vi "Button and Switch CCS.vi"() -> ()   [LabVIEW 2020]
uses:
  <vilib>/addons/control/pid/autopid.llb/PID autotuning parameters (adv).ctl
  <vilib>/addons/control/pid/pid.llb/PID Time Unit.ctl
  <vilib>/addons/control/pid/pid.llb/PID Structure.ctl
  <vilib>/addons/control/pid/pid.llb/PID Gain Unit.ctl
  <vilib>/Instr/_visa.llb/VISA Configure Serial Port (Instr).vi
  <vilib>/addons/control/pid/pid.llb/PID Structure Conversion (DBL).vi
  <vilib>/addons/control/pid/pid.llb/PID Advanced (DBL).vi
  <vilib>/addons/control/pid/NI_PID_autopid.lvlib
  <vilib>/ptbypt/NI_PtbyPt.lvlib
  <vilib>/addons/control/pid/NI_PID_pid.lvlib
panel:
  out "PWM Previous":dbl
  in  "auto? ACC":bool=TRUE
  out "Limit Setpoint":u64
  out "Limit Active":bool
  in  "Limit -":bool
  in  "Limit +":bool
  in  "Limit Speed":bool
  in  "gamma":dbl format="%.2f"
  in  "alpha":dbl=0.2 format="%.2f"
  in  "proportional unit":T1 items=["Gain (K)", "Band (PB)"]
  in  "PID structure":T2 items=["Academic (Standard)", "Parallel", "Series"]
  in  "derivative unit":T3=1 items=["min", "s"]
  in  "integral unit":T3=1 items=["min", "s"]
  in  "derivative":dbl
  in  "integral":dbl
  in  "proportional":dbl=10.0
  in  "linearity":dbl=0.9 format="%.2f"
  in  "beta":dbl=0.7 format="%.2f"
  in  "reinitialize? (F) 2":bool
  out "Speed Setpoint (km/h)":dbl
  out "Target Distance (m)":dbl
  out "Time Level":dbl=1.0
  out "Distance (m)":i8=73
  out "Brake Light":bool
  in  "VISA resource name":refnum<visa-resource-name>="COM15"
  in  "baud rate":u32=115200
  out "RPM":i64(knob) scale=0.0..650.0
  out "VELOCITY":u64(knob) scale=0.0..200.0
  out "GAS PEDAL":u8(slide)=1 scale=0.0..255.0
  out "BRAKE PEDAL":u8(slide)=1 scale=0.0..255.0
  out "VELOCITY":cluster{"VELOCITY":u64, "Cruise Setpoint":u64}(graph)
  in  "autotune? (F)":bool
  in  "PID gains":T4={"proportional gain (Kc)"=0.261831, "integral time (Ti, min)"=0.013639, "derivative time (Td, min)"=0.0} {"derivative time (Td, min)" format="%#.6g"; "integral time (Ti, min)" format="%#.6g"; "proportional gain (Kc)" format="%#.6g"}
  in  "dt (s)":dbl=0.02
  in  "reinitialize? (F)":bool
  in  "autotuning parameters":T5={"technique"=0, "type of controller"=1, "control specification"=0, "amplitude"=30.0} {"amplitude" format="%.2f"; "control specification" items=["normal", "fast", "slow"]; "type of controller" items=["P", "PI", "PID"]; "technique" items=["Step Open Loop", "Step Closed Loop", "Relay", "PID Relay"]}
  out "completed?":bool
  out "tuned PID gains":T4={"proportional gain (Kc)"=0.664899, "integral time (Ti, min)"=0.008397, "derivative time (Td, min)"=0.0} {"derivative time (Td, min)" format="%#.6g"; "integral time (Ti, min)" format="%#.6g"; "proportional gain (Kc)" format="%#.6g"}
  in  "auto? Speed Control":bool
  in  "ACCEPT SPEED PID":bool
  out "MOTOR CONTROL":dbl(graph)=1.0
  in  "stop":bool
  in  "PID Mode":i64(knob)=1 scale=1.0..3.0
  in  "Cruise Enable":bool
  in  "Distance":bool
  out "Distance Level":i8=1
  out "Cruise Active":bool
  out "Cruise Setpoint":u64
  in  "Speed +":bool
  in  "Speed -":bool
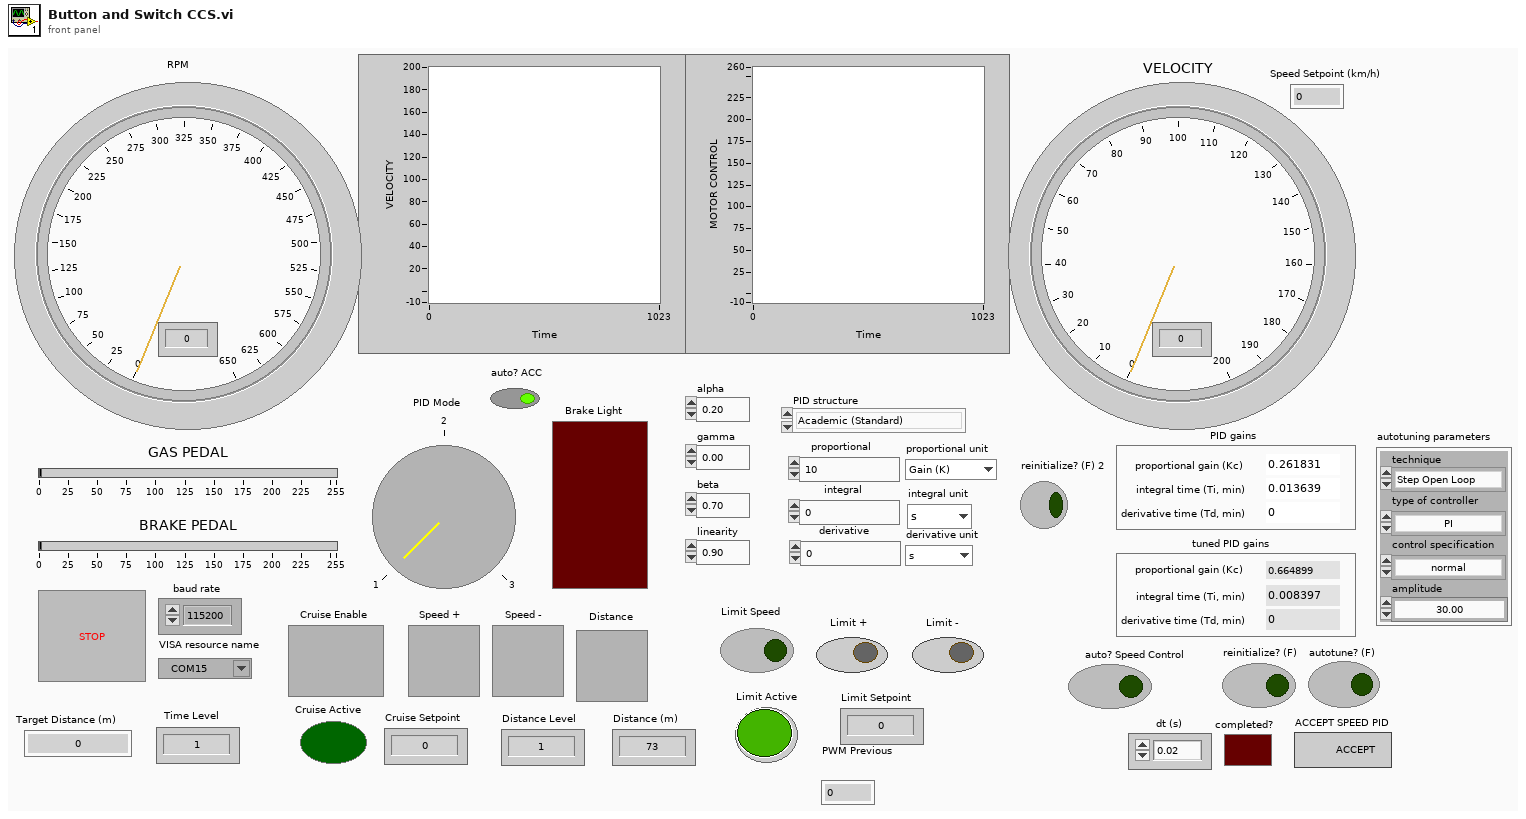
[diagram p1: front panel]
types:
  T1 = typedef "NI_PID_pid.lvlib/PID Gain Unit.ctl" = u16
  T2 = typedef "NI_PID_pid.lvlib/PID Structure.ctl" = u16
  T3 = typedef "NI_PID_pid.lvlib/PID Time Unit.ctl" = u16
  T4 = cluster{"proportional gain (Kc)":dbl, "integral time (Ti, min)":dbl, "derivative time (Td, min)":dbl}
  T5 = typedef "NI_PID_autopid.lvlib/PID autotuning parameters (adv).ctl" = cluster{"technique":u16, "type of controller":u16, "control specification":u16, "amplitude":dbl}
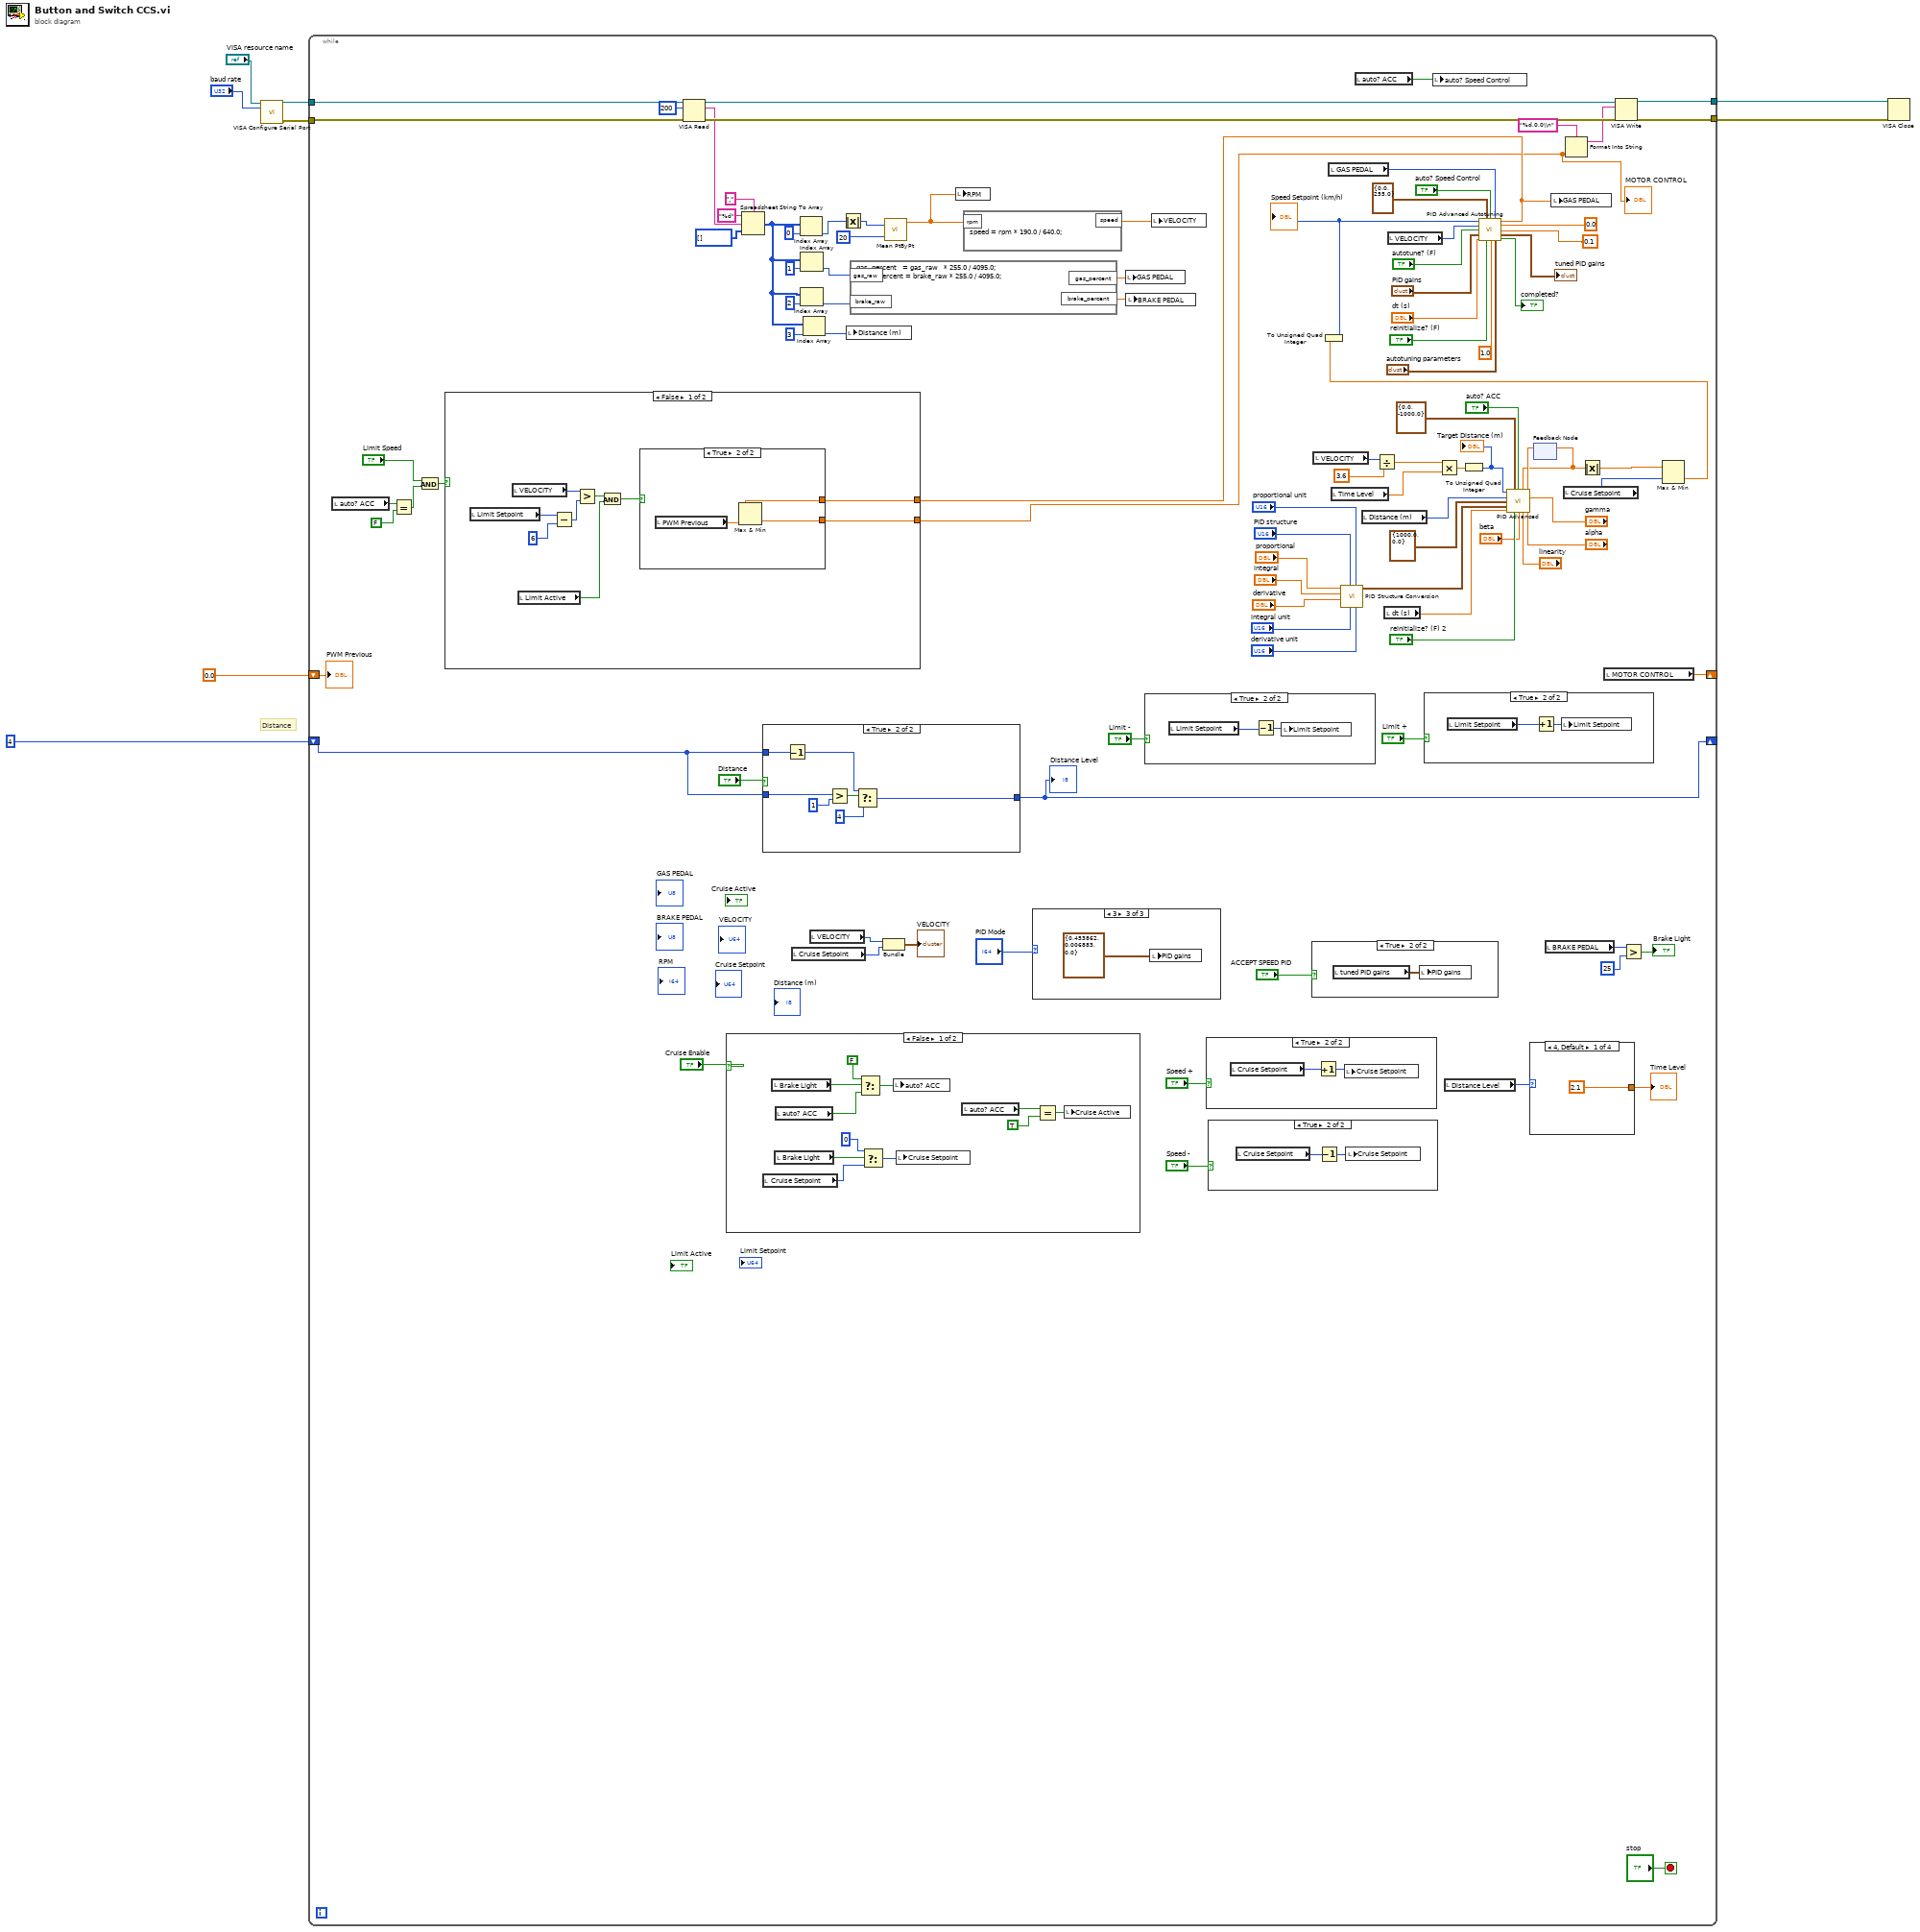
[diagram p0: block diagram]
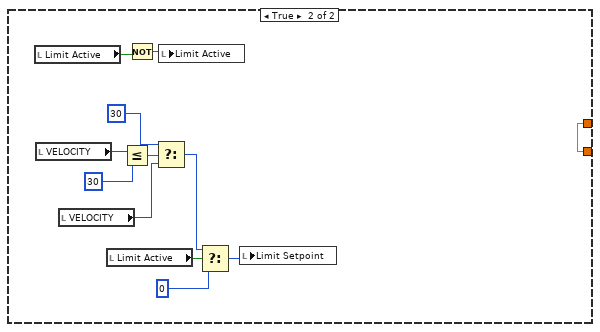
[diagram p5: hidden frame]
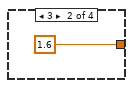
[diagram p6: hidden frame]
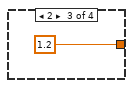
[diagram p7: hidden frame]
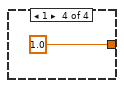
[diagram p8: hidden frame]
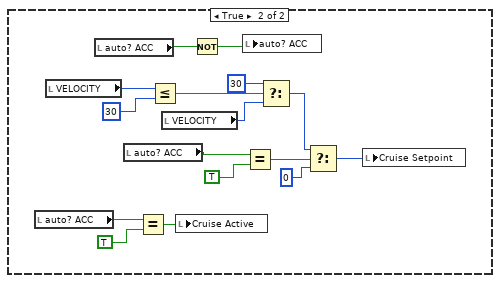
[diagram p12: hidden frame]
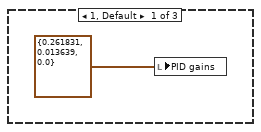
[diagram p13: hidden frame]
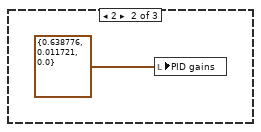
[diagram p14: hidden frame]
diagram:
  # "Distance"
  n1 = call-poly "VISA Configure Serial Port"("VISA resource name"="VISA resource name", "baud rate (9600)"="baud rate") -> ("VISA resource name out"=w7:refnum<visa-resource-name>, "error out"=w6:errorcluster)  [unwired: 12 in]
  n2 = while {
    tunnel: w7 -> [w109]
    tunnel: w6 -> [w108]
    tunnel: [w83] -> w5
    tunnel: [w84] -> w4
    shift-right: [w60] -> _
    shift-left: i64 4 ("f") -> [w61]
    shift-right: [w15] -> _
    shift-left: 0.0 ("MOTOR CONTROL") -> [w13]
    stop <- "stop" stop-if-true
    n3 = local read "auto? ACC"() -> (w20:bool)
    n4 = Equal?(x=w20, y=FALSE) -> (x = y?=w19:bool)
    n5 = And(x="Limit Speed", y=w19) -> (x .and. y?=w12:bool)
    n6 = VISA Read(VISA resource name=w109, byte count=u32 200, error in (no error)=w108) -> (VISA resource name out=w106:refnum<visa-resource-name>, read buffer=w104:string, error out=w107:errorcluster)  [unwired: 1 out]
    n7 = case shown="False" "Cruise Enable" {
      frame False {
        n8 = local read "Cruise Setpoint"() -> (w157:u64)
        n9 = local read "Brake Light"() -> (w165:bool)
        n10 = local read "Brake Light"() -> (w158:bool)
        n11 = local read "auto? ACC"() -> (w162:bool)
        n12 = Select(t=FALSE, s=w165, f=w162) -> (s? t:f=w163:bool)
        n13 = Select(t=u64 0, s=w158, f=w157) -> (s? t:f=w155:u64)
        n14 = local write "auto? ACC"(w163) -> ()
        n15 = local write "Cruise Setpoint"(w155) -> ()
        n16 = local read "auto? ACC"() -> (w160:bool)
        n17 = Equal?(x=w160, y=TRUE) -> (x = y?=w159:bool)
        n18 = local write "Cruise Active"(w159) -> ()
      }
      frame True {
        n19 = local read "auto? ACC"() -> (w173:bool)
        n20 = local read "VELOCITY"() -> (w172:u64)
        n21 = local read "auto? ACC"() -> (w181:bool)
        n22 = local read "auto? ACC"() -> (w179:bool)
        n23 = Equal?(x=w173, y=TRUE) -> (x = y?=w166:bool)
        n24 = Less Or Equal?(x=w172, y=u64 30) -> (x <= y?=w170:bool)
        n25 = local read "VELOCITY"() -> (w169:u64)
        n26 = local write "Cruise Active"(w166) -> ()
        n27 = Not(x=w181) -> (.not. x?=w180:bool)
        n28 = local write "auto? ACC"(w180) -> ()
        n29 = Equal?(x=w179, y=TRUE) -> (x = y?=w177:bool)
        n30 = Select(t=u64 30, s=w170, f=w169) -> (s? t:f=w167:u64)
        n31 = Select(t=w167, s=w177, f=i64 0) -> (s? t:f=w176:u64)
        n32 = local write "Cruise Setpoint"(w176) -> ()
      }
    }
    n33 = Spreadsheet String To Array(delimiter (Tab)=",", format string="%d", spreadsheet string=w104, array type (2D Dbl)=i32[] []) -> (array=w56:i32[])
    n34 = case shown="True" "Distance" {
      tunnel: w61 -> [w143 w150]
      tunnel: w61 -> [_ w149]
      tunnel: [w143 w144] -> w60
      frame False {
      }
      frame True {
        n35 = Decrement(x=w150) -> (x-1=w146:i64)
        n36 = Greater?(x=w149, y=i64 1) -> (0:w147:bool)
        n37 = Select(t=w146, s=w147, f=i64 4) -> (s? t:f=w144:i64)
      }
    }
    "Distance Level" <- w60
    n38 = local read "Cruise Setpoint"() -> (w65:u64)
    n39 = Index Array(array=w56, index=0) -> (element=w77:i32)
    n40 = Index Array(array=w56, index=1) -> (element=w80:i32)
    n41 = Index Array(array=w56, index=2) -> (element=w79:i32)
    n42 = Index Array(array=w56, index=3) -> (element=w54:i32)
    n43 = local read "VELOCITY"() -> (w72:u64)
    n44 = Absolute Value(x=w77) -> (abs(x)=w76:i32)
    n45 = local write "Distance (m)"(w54) -> ()
    n46 = formula code="gas_percent   = gas_raw   * 255.0 / 4095.0;\nbrake_percent = brake_raw * 255.0 / 4095.0;"("gas_raw"=w80, "brake_raw"=w79) -> ("gas_percent"=w10:dbl, "brake_percent"=w78:dbl)
    n47 = Bundle("VELOCITY"=w72, "Cruise Setpoint"=w65) -> (→"VELOCITY":cluster{"VELOCITY":u64, "Cruise Setpoint":u64})  [unwired: 1 in]
    n48 = call <vilib>:"Mean PtByPt.vi"("x"=w76, "sample length"=20) -> ("mean"=w81:dbl)  [unwired: 2 in, 1 out]
    n49 = local write "RPM"(w81) -> ()
    n50 = formula code="speed = rpm * 190.0 / 640.0;"("rpm"=w81) -> ("speed"=w82:dbl)
    n51 = case shown="3" "PID Mode" {
      frame 1, Default {
        n52 = local write "PID gains"(T4 {"proportional gain (Kc)"=0.261831, "integral time (Ti, min)"=0.013639, "derivative time (Td, min)"=0.0} ("PID gains")) -> ()
      }
      frame 2 {
        n53 = local write "PID gains"(T4 {"proportional gain (Kc)"=0.638776, "integral time (Ti, min)"=0.011721, "derivative time (Td, min)"=0.0} ("PID gains")) -> ()
      }
      frame 3 {
        n54 = local write "PID gains"(T4 {"proportional gain (Kc)"=0.453862, "integral time (Ti, min)"=0.006883, "derivative time (Td, min)"=0.0} ("PID gains")) -> ()
      }
    }
    n55 = local write "GAS PEDAL"(w10) -> ()
    n56 = local write "BRAKE PEDAL"(w78) -> ()
    n57 = case shown="True" "Limit -" {
      frame False {
      }
      frame True {
        n58 = local read "Limit Setpoint"() -> (w111:u64)
        n59 = Decrement(x=w111) -> (x-1=w110:u64)
        n60 = local write "Limit Setpoint"(w110) -> ()
      }
    }
    n61 = local write "VELOCITY"(w82) -> ()
    n62 = case shown="True" "Speed +" {
      frame False {
      }
      frame True {
        n63 = local read "Cruise Setpoint"() -> (w153:u64)
        n64 = Increment(x=w153) -> (x+1=w154:u64)
        n65 = local write "Cruise Setpoint"(w154) -> ()
      }
    }
    n66 = case shown="True" "Speed -" {
      frame False {
      }
      frame True {
        n67 = local read "Cruise Setpoint"() -> (w152:u64)
        n68 = Decrement(x=w152) -> (x-1=w151:u64)
        n69 = local write "Cruise Setpoint"(w151) -> ()
      }
    }
    n70 = case shown="True" "ACCEPT SPEED PID" {
      frame False {
      }
      frame True {
        n71 = local read "tuned PID gains"() -> (w185:T4)
        n72 = local write "PID gains"(w185) -> ()
      }
    }
    n73 = local read "VELOCITY"() -> (w48:u64)
    n74 = local read "GAS PEDAL"() -> (w67:u8)
    n75 = local read "Time Level"() -> (w49:dbl)
    n76 = call-poly <vilib>:"PID Structure Conversion.vi"("derivative unit"="derivative unit", "proportional unit"="proportional unit", "integral unit"="integral unit", "PID structure"="PID structure", "derivative"="derivative", "integral"="integral", "proportional"="proportional") -> ("PID gains"=w25:T4)  [unwired: 4 in]
    n77 = local read "auto? ACC"() -> (w21:bool)
    n78 = local read "Distance (m)"() -> (w47:i8)
    n79 = Divide(x=w48, y=3.6) -> (x/y=w50:dbl)
    n80 = local read "dt (s)"() -> (w41:dbl)
    n81 = local read "VELOCITY"() -> (w95:u64)
    n82 = case shown="True" "Limit +" {
      frame False {
      }
      frame True {
        n83 = local read "Limit Setpoint"() -> (w113:u64)
        n84 = Increment(x=w113) -> (x+1=w112:u64)
        n85 = local write "Limit Setpoint"(w112) -> ()
      }
    }
    n86 = local write "auto? Speed Control"(w21) -> ()
    n87 = Multiply(x=w50, y=w49) -> (x*y=w36:dbl)
    n88 = local read "Distance Level"() -> (w53:i8)
    n89 = To Unsigned Quad Integer(1:w36) -> (0:w35:u64)
    "Target Distance (m)" <- w35
    n90 = case shown="4, Default" w53 {
      tunnel: [2.1 ("Time Level") 1.6 ("Time Level") 1.2 ("Time Level") 1.0 ("Time Level")] -> w52
      frame 4, Default {
      }
      frame 3 {
      }
      frame 2 {
      }
      frame 1 {
      }
    }
    "Time Level" <- w52
    n91 = feedback #1() -> (w40:dbl)  [unwired: 1 in]
    n92 = call-poly <vilib>:"PID Advanced.vi"("setpoint"=w35, "output range"=cluster{"output high":dbl, "output low":dbl} {"output high"=0.0, "output low"=-1000.0}, "auto? (T)"="auto? ACC", "manual control"=w40, "process variable"=w47, "gamma"="gamma", "setpoint range"=cluster{"setpoint high":dbl, "setpoint low":dbl} {"setpoint high"=1000.0, "setpoint low"=0.0}, "alpha"="alpha", "PID gains"=w25, "dt (s)"=w41, "reinitialize? (F)"="reinitialize? (F) 2", "beta"="beta", "linearity"="linearity") -> ("output"=w42:dbl)  [unwired: 1 in, 1 out]
    n93 = feedback-in #1(w42) -> ()
    n94 = local read "BRAKE PEDAL"() -> (w59:u8)
    n95 = local read "Cruise Setpoint"() -> (w44:u64)
    n96 = Absolute Value(x=w40) -> (abs(x)=w39:dbl)
    n97 = local read "MOTOR CONTROL"() -> (w15:dbl)
    n98 = Greater?(x=w59, y=u8 25) -> (0:→"Brake Light":bool)
    n99 = Max & Min(x=w39, y=w44) -> (min(x,y)=w33:dbl)  [unwired: 1 out]
    n100 = To Unsigned Quad Integer(1:w33) -> (0:w34:u64)
    "Speed Setpoint (km/h)" <- w34
    n101 = call <vilib>:"PID Advanced Autotuning.vi"("setpoint"=w34, "output range"=cluster{"output high":dbl, "output low":dbl} {"output high"=0.0, "output low"=255.0}, "auto? (F)"="auto? Speed Control", "manual control"=w67, "process variable"=w95, "gamma"=0.0, "autotune? (F)"="autotune? (F)", "alpha"=0.1, "PID gains"="PID gains", "dt (s)"="dt (s)", "reinitialize? (F)"="reinitialize? (F)", "beta"=1.0, "autotuning parameters"="autotuning parameters") -> ("output"=w11:dbl, "tuned PID gains"=→"tuned PID gains":T4, "tuning completed?"=→"completed?":bool)
    n102 = case shown="False" w12 {
      tunnel: w11 -> [w121 w127]
      tunnel: [w120 w127] -> w9
      frame False {
        n103 = local read "Limit Setpoint"() -> (w115:u64)
        n104 = local read "VELOCITY"() -> (w122:u64)
        n105 = local read "Limit Active"() -> (w118:bool)
        n106 = Subtract(x=w115, y=u64 6) -> (x-y=w116:u64)
        n107 = Greater?(x=w122, y=w116) -> (0:w119:bool)
        n108 = And(x=w119, y=w118) -> (x .and. y?=w117:bool)
        n109 = case shown="True" w117 {
          tunnel: w121 -> [w123 w125]
          tunnel: [w123 w124] -> w120
          frame False {
          }
          frame True {
            n110 = local read "PWM Previous"() -> (w126:dbl)
            n111 = Max & Min(x=w125, y=w126) -> (min(x,y)=w124:dbl)  [unwired: 1 out]
          }
        }
      }
      frame True {
        n112 = local read "Limit Active"() -> (w132:bool)
        n113 = local read "VELOCITY"() -> (w138:u64)
        n114 = local read "VELOCITY"() -> (w135:u64)
        n115 = local read "Limit Active"() -> (w131:bool)
        n116 = Less Or Equal?(x=w138, y=u64 30) -> (x <= y?=w136:bool)
        n117 = Not(x=w132) -> (.not. x?=w133:bool)
        n118 = Select(t=u64 30, s=w136, f=w135) -> (s? t:f=w130:u64)
        n119 = local write "Limit Active"(w133) -> ()
        n120 = Select(t=w130, s=w131, f=u64 0) -> (s? t:f=w128:u64)
        n121 = local write "Limit Setpoint"(w128) -> ()
      }
    }
    "MOTOR CONTROL" <- w9
    n122 = local write "GAS PEDAL"(w11) -> ()
    n123 = Format Into String(format string="%d,0,0\\n", w9) -> (resulting string=w96:string)  [unwired: 2 in, 1 out]
    n124 = VISA Write(VISA resource name=w106, write buffer=w96, error in (no error)=w107) -> (VISA resource name out=w84:refnum<visa-resource-name>, error out=w83:errorcluster)  [unwired: 1 out]
    "PWM Previous" <- w13
  }
  n125 = VISA Close(VISA resource name=w4, error in (no error)=w5) -> ()  [unwired: 1 out]
